vi "GetTunnelIndexing.vi"(5 "Tunnel in":refnum<class "Tunnel.lvclass">, 6 "error in":errorcluster, 9 "VI Interpreter in":refnum<class "VI Interpreter.lvclass">) -> (0 "error out":errorcluster, 3 "VI Interpreter out":refnum<class "VI Interpreter.lvclass">, 4 "Tunnel out":refnum<class "Tunnel.lvclass">)   [LabVIEW 2014, in "VI Interpreter.lvclass"]
uses:
  VI Interpreter.lvclass
  Tunnel/Tunnel.lvclass
  LoopTunnel/LoopTunnel.lvclass
  LoopTunnel/LoopTunnel.lvclass/LoopTunnel.ctl
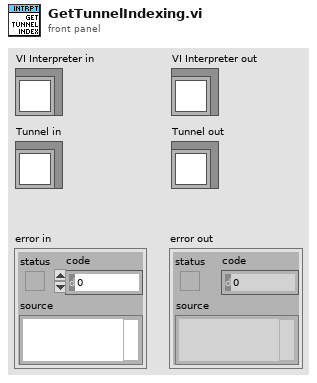
[diagram p1: front panel]
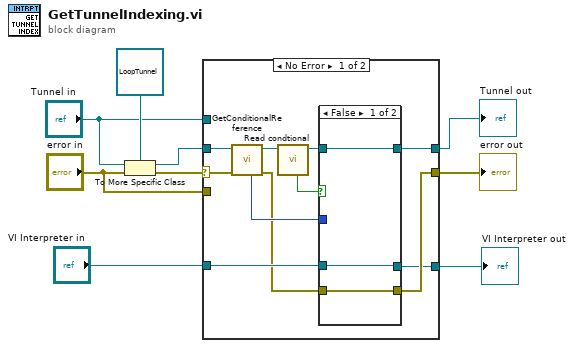
[diagram p0: block diagram]
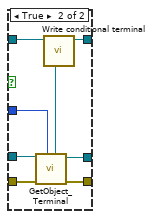
[diagram p2: hidden frame]
diagram:
  n1 = To More Specific Class(target class=refnum<class "LoopTunnel.lvclass"> refnum ("LoopTunnel.lvclass"), reference="Tunnel in", error in="error in") -> (specific class reference=w7:refnum<class "LoopTunnel.lvclass">, error out=w8:errorcluster)
  n2 = case shown="No Error" w8 {
    selector: w8 -> [w19 _]
    tunnel: w7 -> [w20 _]
    tunnel: "Tunnel in" -> [_ w33]
    tunnel: [w14 w34] -> w2
    tunnel: [w16 w33] -> w3
    tunnel: "error in" -> [_ w34]
    tunnel: "VI Interpreter in" -> [w18 w32]
    tunnel: [w13 w32] -> w1
    frame No Error {
      n3 = call "GetConditionalReference.vi"("error in"=w19, "LoopTunnel in"=w20) -> ("error out"=w15:errorcluster, "LoopTunnel out"=w12:refnum<class "LoopTunnel.lvclass">, "UID"=w17:i32)  [unwired: 5 in]
      n4 = call "Read condtional.vi"("LoopTunnel in"=w12) -> ("LoopTunnel out"=w11:refnum<class "LoopTunnel.lvclass">, "condtional"=w10:bool)  [unwired: 7 in]
      n5 = case shown="False" w10 {
        tunnel: w18 -> [w21 w31]
        tunnel: w17 -> [_ w30]
        tunnel: [w23 w29] -> w16
        tunnel: w15 -> [w22 w27]
        tunnel: [w22 w26] -> w14
        tunnel: [w21 w25] -> w13
        tunnel: w11 -> [w23 w24]
        frame False {
        }
        frame True {
          n6 = call "GetObject_Terminal.vi"("UID"=w30, "error in"=w27, "VI Interpreter in"=w31) -> ("error out"=w26:errorcluster, "VI Interpreter out"=w25:refnum<class "VI Interpreter.lvclass">, "Terminal"=w28:refnum<class "Terminal.lvclass">)  [unwired: 3 in, 1 out]
          n7 = call "Write conditional terminal.vi"("conditional terminal"=w28, "LoopTunnel in"=w24) -> ("LoopTunnel out"=w29:refnum<class "LoopTunnel.lvclass">)  [unwired: 7 in]
        }
      }
    }
    frame Error {
    }
  }
  "error out" <- w2
  "VI Interpreter out" <- w1
  "Tunnel out" <- w3
